vi "Get Inspection Data.vi"(8 "error in (no error)":errorcluster, 10 "program names":string[](array[string]), 11 "IPF sub folders":path[](array[path])) -> (0 "error out":errorcluster, 2 "IPF sub folders":path[](array[path]), 3 "Inspection Data":T1[](array[typedef]))   [LabVIEW 2013]
uses:
  3013/code/Modules/GUI/GUI_5/subPanels/program/type_def/Inspection program data.ctl
  3013/code/Modules/Configuration/type_def/Scan Params.ctl
  3013/code/Modules/Configuration/type_def/Profile Resolution.ctl
  3013/code/Modules/Preprocess Data/type_def/direction.ctl
  3013/code/Modules/Inspection/Data/Panel_class/type_def/Control file rel path.ctl
  3013/code/Modules/GUI/GUI_5/subPanels/edit/type_def/Description.ctl
  type_def/files.ctl
  3013/code/Modules/Inspection/Data/Panel_class/type_def/Config File data.ctl
  3013/code/Modules/Inspection/type_def/Pos and Rot.ctl
  3013/code/Modules/Inspection/Data/PCB_class/type_def/PCB Params.ctl
  3013/code/Modules/Inspection/Data/Panel_class/type_def/BarCode Params.ctl
  3013/code/Modules/Barcode Reader/type_def/id.ctl
  <userlib>/_OpenG.lib/file/file.llb/File Exists - Scalar__ogtk.vi
  3013/code/Modules/Configuration/Config.lvlib
  3013/code/Modules/GUI/GUI_5/subPanels/program/program.lvlib
  3013/code/Modules/Inspection/Data/Panel_class/Panel.lvclass
  3013/code/Modules/Preprocess Data/PreProcess.lvlib
  <vilib>/Utility/config.llb/NI_LVConfig.lvlib
  3013/code/Modules/Inspection/Inspection.lvlib
  3013/code/Modules/Inspection/Data/PCB_class/PCB.lvclass
  3013/code/Modules/Barcode Reader/Barcode Reader.lvlib
  a3Di APG.lvlib
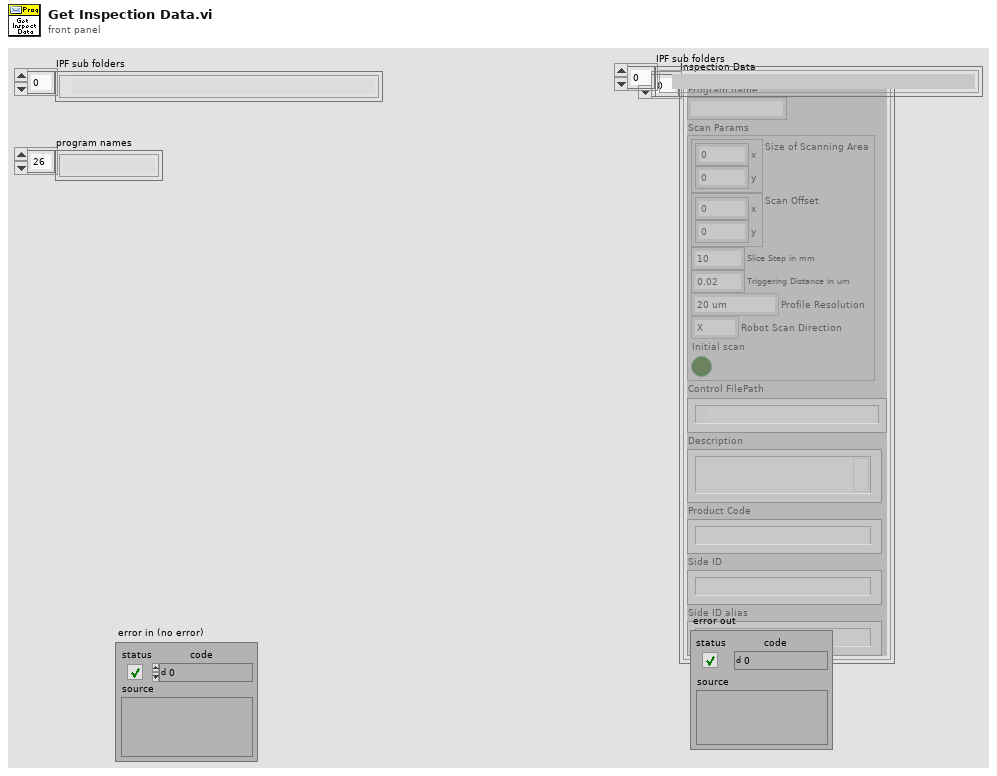
[diagram p1: front panel]
types:
  T1 = typedef "GUI.lvlib/subPanel.lvlib/program.lvlib/Inspection program data.ctl" = cluster{"Program name":string, "Scan Params":T2, "Control FilePath":T5, "Description":T6, "Product Code":T6, "Side ID":T6, "Side ID alias":T6}
  T2 = typedef "Config.lvlib/Scan Params.ctl" = cluster{"Size of Scanning Area":cluster{"x":dbl, "y":dbl}, "Scan Offset":cluster{"x":dbl, "y":dbl}, "Slice Step in mm":dbl, "Triggering Distance in mm":dbl, "Triggering Distance in um":dbl, "Profile Resolution":T3, "Version":string, "Robot Scan Direction":T4, "Initial scan":bool}
  T3 = typedef "Config.lvlib/Profile Resolution.ctl" = enum8{"20 um", "40 um"}
  T4 = typedef "PreProcess.lvlib/direction.ctl" = enum8{"X", "Y"}
  T5 = typedef "Inspection.lvlib/Panel.lvclass/Control file rel path.ctl" = path
  T6 = typedef "Description.ctl" = string
  T7 = typedef "a3Di APG.lvlib/files.ctl" = cluster{"Programming Files":cluster{"PCB Design Identity":string, "ODB++ file":path, "Result temp  folder":path, "IPF temp folder":path}, "ODB file Converted?":bool, "Panel Params":T8, "PCB Outline File":path, "Initial Scan":bool, "PCBs on a carrier":bool, "Carrier Size":cluster{"X":dbl, "Y":dbl}, "IPF modified":bool, "PCB Side":enum16{"Top", "Bottom"}}
  T8 = typedef "Inspection.lvlib/Panel.lvclass/Config File data.ctl" = cluster{"Name":string, "Pos & Rot":T9, "PCBs List":cluster{"PCB Params":T10}[], "PCB BarCode Params":T11[], "Scan Type":bool}
  T9 = typedef "Inspection.lvlib/Pos and Rot.ctl" = cluster{"X":dbl, "Y":dbl, "Z":dbl, "rotation":dbl}
  T10 = typedef "Inspection.lvlib/PCB.lvclass/PCB Params.ctl" = cluster{"Name":string, "Pos & Rot":T9}
  T11 = typedef "Inspection.lvlib/Panel.lvclass/BarCode Params.ctl" = cluster{"ID":T12}
  T12 = typedef "Barcode Reader.lvlib/id.ctl" = u8
  T13 = typedef "NI_LVConfig.lvlib/Config Data RefNum.ctl" = refnum<k1>
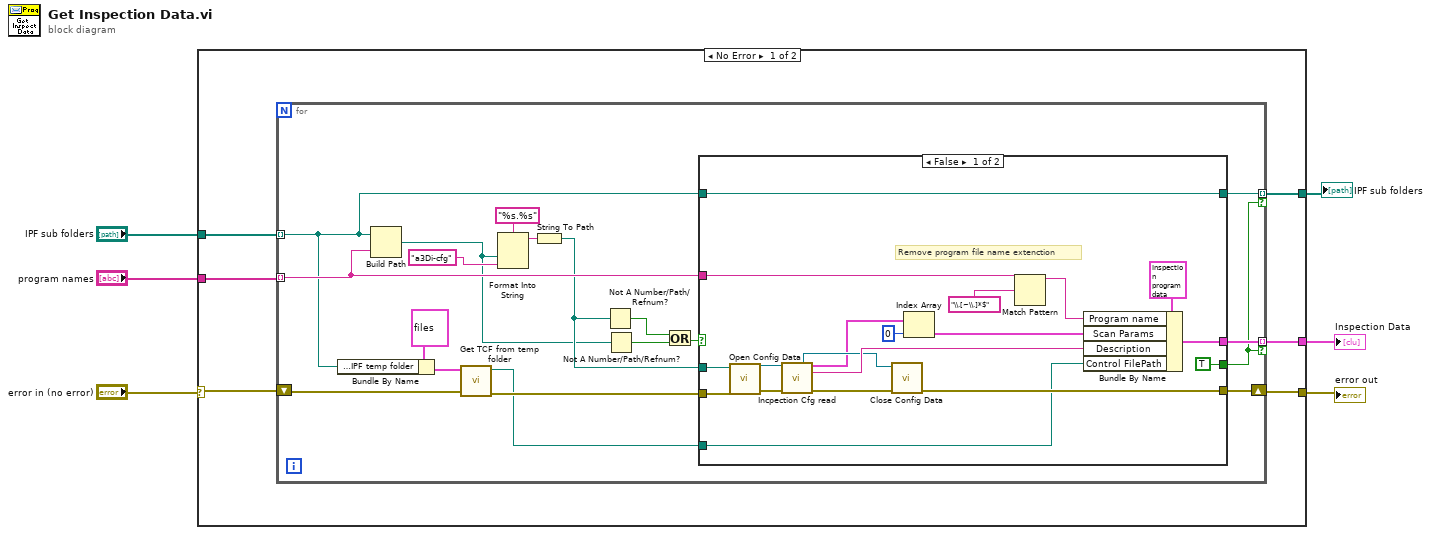
[diagram p0: block diagram]
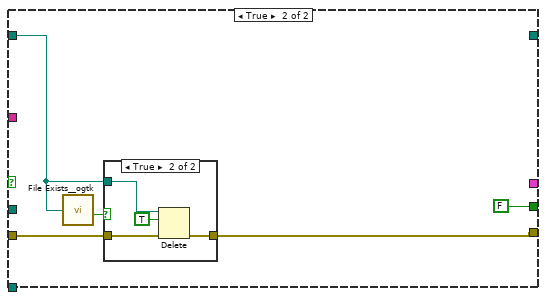
[diagram p2: hidden frame]
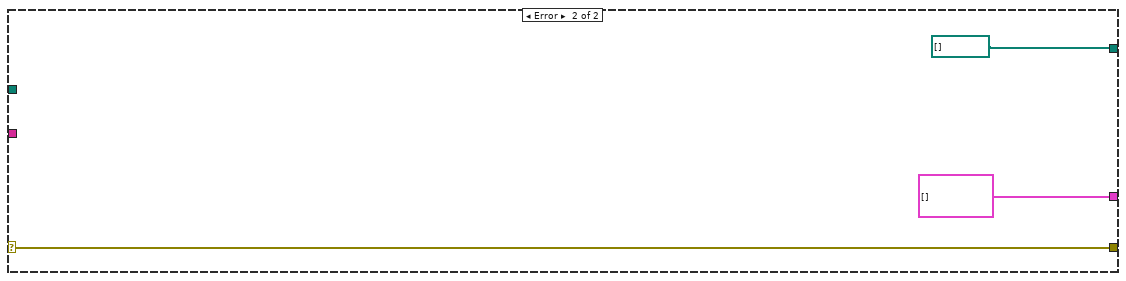
[diagram p4: hidden frame]
diagram:
  n1 = case shown="No Error" "error in (no error)" {
    selector: "error in (no error)" -> [w10 w63]
    tunnel: [w12 w63] -> w5
    tunnel: [w11 T1[] []] -> w4
    tunnel: "IPF sub folders" -> [w9 _]
    tunnel: "program names" -> [w8 _]
    tunnel: [w7 path[] []] -> w1
    frame No Error {
      n2 = for {
        tunnel: w8 -> [w30] mode=indexing
        tunnel: w9 -> [w16] mode=indexing
        shift-right: [w29] -> w12
        shift-left: w10 -> [w26]
        tunnel: [w31] -> w11 mode=indexing if=w22
        tunnel: [w23] -> w7 mode=indexing if=w22
        n3 = Bundle By Name(cluster=T7 {"Programming Files"={"PCB Design Identity"="", "ODB++ file"=path "Z:/86636871-01-sp.tgz", "Result temp  folder"=path "", "IPF temp folder"=path "C:/Users/admin/AppData/Local/Temp/a3Di/APG/IPF/RR_top_1"}, "ODB file Converted?"=FALSE, "Panel Params"={"Name"="", "Pos & Rot"={"X"=0.0, "Y"=0.0, "Z"=0.0, "rotation"=0.0}, "PCBs List"=[], "PCB BarCode Params"=[], "Scan Type"=FALSE}, "PCB Outline File"=path "", "Initial Scan"=FALSE, "PCBs on a carrier"=FALSE, "Carrier Size"={"X"=0.0, "Y"=0.0}, "IPF modified"=FALSE, "PCB Side"=enum."Top"} ("Programming Data"), "Programming Files.IPF temp folder"=w16) -> (w27:T7)
        n4 = Build Path(base path=w16, name or relative path=w30) -> (appended path=w15:path)
        n5 = call "Get TCF from temp folder.vi"("error in (no error)"=w26, "Programming Data"=w27) -> ("error out"=w25:errorcluster, "TCF file"=w24:path)  [unwired: 8 in]
        n6 = Format Into String(format string="%s.%s", w15, "a3Di-cfg" ("new ending (none)")) -> (resulting string=w19:string)  [unwired: 2 in, 1 out]
        n7 = String To Path(string=w19) -> (path=w20:path)
        n8 = Not A Number/Path/Refnum?(number/path/refnum=w20) -> (NaN/Path/Refnum?=w13:bool)
        n9 = Not A Number/Path/Refnum?(number/path/refnum=w15) -> (NaN/Path/Refnum?=w14:bool)
        n10 = Or(x=w13, y=w14) -> (x .or. y?=w17:bool)
        n11 = case shown="False" w17 {
          tunnel: [w50 _] -> w31
          tunnel: w30 -> [w49 _]
          tunnel: [w40 w53] -> w29
          tunnel: w25 -> [w37 w54]
          tunnel: w24 -> [w36 _]
          tunnel: w20 -> [w34 _]
          tunnel: [TRUE FALSE] -> w22
          tunnel: w16 -> [w32 w51]
          tunnel: [w32 _] -> w23
          frame False {
            # "Remove program file name extenction"
            n12 = call <vilib>:"Open Config Data.vi"("error in (no error)"=w37, "configuration file path"=w34) -> ("error out"=w43:errorcluster, "refnum"=w44:T13)  [unwired: 7 in, 1 out]
            n13 = call "Incpection Cfg read.vi"("Inspection cfg file refnum in"=w44, "error in (no error)"=w43) -> ("Inspection cfg file refnum out"=w38:T13, "Scan Params[]"=w35:T2[], "Description"=w46:T6, "error out"=w39:errorcluster)  [unwired: 7 in, 3 out]
            n14 = call <vilib>:"Close Config Data.vi"("error in (no error)"=w39, "refnum"=w38) -> ("error out"=w40:errorcluster)  [unwired: 8 in, 1 out]
            n15 = Index Array(array=w35, index=0) -> (element=w42:T2)
            n16 = Match Pattern(string=w49, regular expression="\\.[~\\.]*$") -> (before substring=w48:string)  [unwired: 4 out]
            n17 = Bundle By Name(cluster=T1 {"Program name"="", "Scan Params"={"Size of Scanning Area"={"x"=0.0, "y"=0.0}, "Scan Offset"={"x"=0.0, "y"=0.0}, "Slice Step in mm"=0.0, "Triggering Distance in mm"=0.0, "Triggering Distance in um"=0.0, "Profile Resolution"=enum."20 um", "Version"="", "Robot Scan Direction"=enum."X", "Initial scan"=FALSE}, "Control FilePath"=path "", "Description"="", "Product Code"="", "Side ID"="", "Side ID alias"=""}, "Program name"=w48, "Scan Params"=w42, "Description"=w46, "Control FilePath"=w36) -> (w50:T1)
          }
          frame True {
            n18 = call-poly <userlib>:"File Exists__ogtk.vi"("file path"=w51) -> ("exists"=w52:bool)  [unwired: 6 in, 1 out]
            n19 = case shown="True" w52 {
              tunnel: w54 -> [w56 w60]
              tunnel: [w56 w59] -> w53
              tunnel: w51 -> [_ w57]
              frame False {
              }
              frame True {
                n20 = Delete(path (use dialog)=w57, entire hierarchy (F)=TRUE, error in=w60) -> (error out=w59:errorcluster)  [unwired: 2 in, 2 out]
              }
            }
          }
        }
      }
    }
    frame Error {
    }
  }
  "error out" <- w5
  "Inspection Data" <- w4
  "IPF sub folders" <- w1
